vi "Remove Max Setpoints.vi"(8 "error in (no error)":errorcluster, 11 "Calibration Points in":T1[](array[typedef])) -> (0 "error out":errorcluster, 3 "Calibration Points out":T1[](array[typedef]))   [LabVIEW 2026, in "Analysis.lvlib"]
uses:
  controls/Messaging Payloads/Calibration Point Table Insert.ctl
  Analysis.lvlib
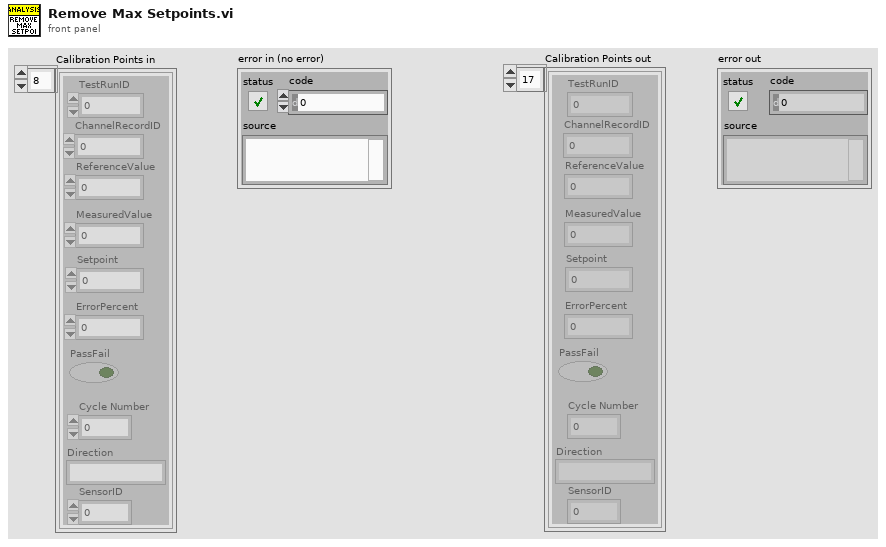
[diagram p1: front panel]
types:
  T1 = typedef "Calibration Point Table Insert.ctl" = cluster{"TestRunID":i32, "ChannelRecordID":i32, "Setpoint":dbl, "MeasuredValue":dbl, "ErrorPercent":dbl, "PassFail":bool, "ReferenceValue":dbl, "Cycle Number":i32, "Direction":string, "SensorID":i32}
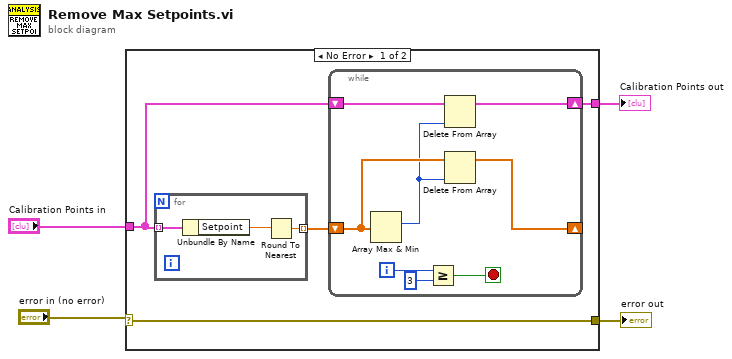
[diagram p0: block diagram]
diagram:
  n1 = case shown="No Error" "error in (no error)" {
    selector: "error in (no error)" -> [w5 w21]
    tunnel: "Calibration Points in" -> [w7 w20]
    tunnel: [w6 w20] -> w3
    tunnel: [w5 w21] -> w1
    frame No Error {
      n2 = for {
        tunnel: w7 -> [w19] mode=indexing
        tunnel: [w17] -> w8 mode=indexing
        n3 = Unbundle By Name(w19) -> ("Setpoint"=w18:dbl)
        n4 = Round To Nearest(number=w18) -> (nearest integer value=w17:dbl)
      }
      n5 = while {
        shift-right: [w15] -> _
        shift-left: w8 -> [w16]
        shift-right: [w9] -> w6
        shift-left: w7 -> [w11]
        i -> [w14]
        stop <- w12 stop-if-true
        n6 = Array Max & Min(array=w16) -> (max index (indices)=w10:i32)  [unwired: 3 out]
        n7 = Greater Or Equal?(x=w14, y=3) -> (x >= y?=w12:bool)
        n8 = Delete From Array(array=w11, index=w10) -> (array with subset deleted=w9:T1[])  [unwired: 1 in, 1 out]
        n9 = Delete From Array(array=w16, index=w10) -> (array with subset deleted=w15:dbl[])  [unwired: 1 in, 1 out]
      }
    }
    frame Error {
    }
  }
  "Calibration Points out" <- w3
  "error out" <- w1
